vi "Synchronize Triggers.vi"(7 "Reset":bool, 10 "In2":bool, 11 "In1":bool) -> (3 "Out":bool)   [LabVIEW 2014]
panel:
  # "Copyright 2014 Vidrio Technologies\nScanImage 5 software is licensed under the Apache License, Version 2.0 (the \"License\"); you may not use any files contained\nwithin the ScanImage 5 release except in compliance with the License. You may obtain a copy of the License at\n http://www.apache.org/licenses/LICENSE-2.0\nUnless required by applicable law or agreed to in writing, software distributed under the License is distributed on an\n\"AS IS\" BASIS, WITHOUT WARRANTIES OR CONDITIONS OF ANY KIND, either express or implied. See the License for the\n specific language governing permissions and limitations under the License."
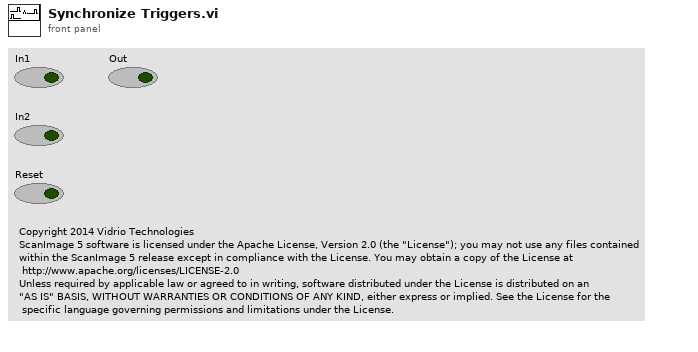
[diagram p1: front panel]
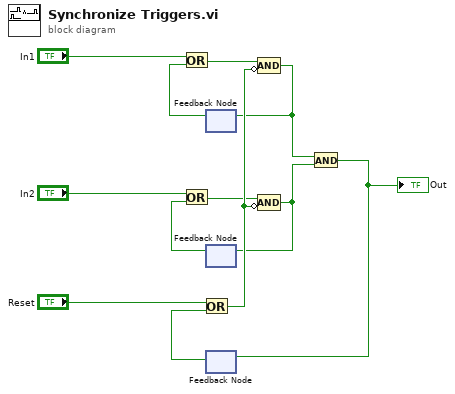
[diagram p0: block diagram]
diagram:
  n1 = feedback #1() -> (w2:bool)  [unwired: 1 in]
  n2 = Or(x="In1", y=w2) -> (x .or. y?=w3:bool)
  n3 = feedback #2() -> (w5:bool)  [unwired: 1 in]
  n4 = Or(x="In2", y=w5) -> (x .or. y?=w4:bool)
  n5 = feedback #3() -> (w10:bool)  [unwired: 1 in]
  n6 = Or(x="Reset", y=w10) -> (x .or. y?=w11:bool)
  n7 = Compound Arithmetic op=AND(w3, invert w11) -> (w7:bool)
  n8 = feedback-in #1(w7) -> ()
  n9 = Compound Arithmetic op=AND(w4, invert w11) -> (w8:bool)
  n10 = feedback-in #2(w8) -> ()
  n11 = And(x=w7, y=w8) -> (x .and. y?=w9:bool)
  "Out" <- w9
  n12 = feedback-in #3(w9) -> ()
